vi "Average6.vi"() -> ()   [LabVIEW 2016]
panel:
  in  "6":dbl
  in  "5":dbl format="%#_13g"
  out "average":dbl
  in  "4":dbl
  in  "3":dbl
  in  "2":dbl
  in  "1":dbl
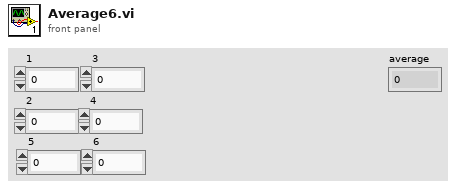
[diagram p1: front panel]
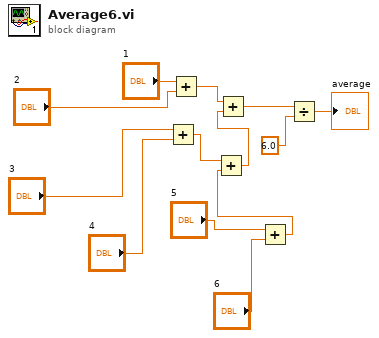
[diagram p0: block diagram]
diagram:
  n1 = Add(x="3", y="4") -> (x+y=w5:dbl)
  n2 = Add(x="1", y="2") -> (x+y=w13:dbl)
  n3 = Add(x="5", y="6") -> (x+y=w2:dbl)
  n4 = Add(x=w5, y=w2) -> (x+y=w4:dbl)
  n5 = Add(x=w13, y=w4) -> (x+y=w6:dbl)
  n6 = Divide(x=w6, y=6.0) -> (x/y=→"average":dbl)
